vi "Untitled.vi"() -> ()   [LabVIEW 2010]
uses:
  <instrlib>/niSync/niSync.llb/niSync Initialize (IVI).vi
  glob1.vi
panel:
  out "Timing:Time Reference:Last Synchronization ID":i32
  out "Timing:Time Reference:Clock Resolution":i32
  out "Timing:Time Reference:UTC Offset Valid":bool
  out "Timing:Time Reference:UTC Offset":i32
  out "Timing:Time Reference:Time Reference Correction":dbl
  out "Timing:Time Reference:Offset from Time Reference":dbl
  out "Timing:Time Reference:Is Time Reference Present":bool
  out "Timing:Time Reference:Time Reference":i32(ring) items=["GPS", "IRIG", "PPS", "1588 Ordinary Clock", "Free Running"]
  in  "stop":bool
  out "error out":errorcluster {"code" format="%.0x"}
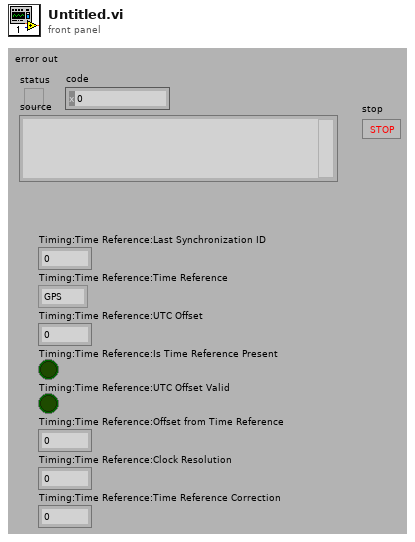
[diagram p1: front panel]
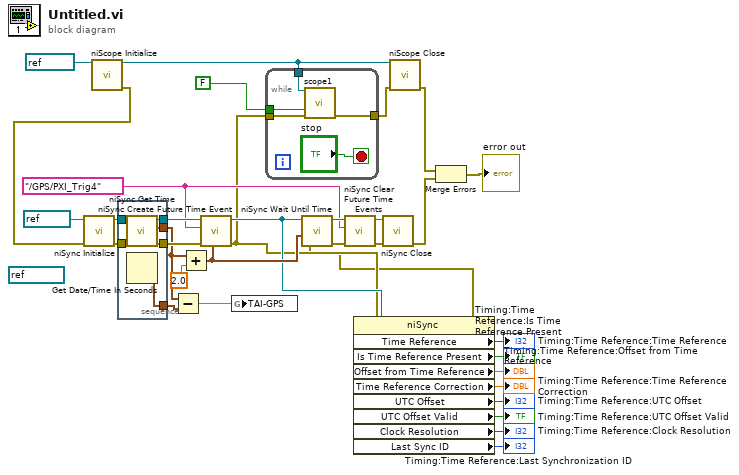
[diagram p0: block diagram]
diagram:
  w26 = tag "/GPS/PXI_Trig4" ("terminal")
  (unwired) refnum<visa-resource-name> "t6682"
  n1 = call <instrlib>:"niScope Initialize.vi"("resource name"=refnum<k15> "ADC") -> ("instrument handle"=w18:refnum<k15>, "error out"=w16:errorcluster)  [unwired: 13 in]
  n2 = call-poly <instrlib>:"niSync Initialize.vi"("error in (no error)"=w16, "resource name"=refnum<k15> "GPS") -> ("error out"=w33:errorcluster, "instrument handle out"=w34:refnum<k15>)  [unwired: 8 in]
  n3 = stacked-sequence {
    tunnel: w34 -> [w40]
    tunnel: w33 -> [w39]
    tunnel: [w38] -> w30
    tunnel: [w37] -> w29
    tunnel: [w36] -> w15
    tunnel: [w35] -> w14
    frame #0 {
      n4 = call <instrlib>:"niSync Get Time.vi"("error in (no error)"=w39, "instrument handle"=w40) -> ("error out"=w38:errorcluster, "time"=w35:timestamp, "instrument handle out"=w37:refnum<k15>)  [unwired: 5 in]
      n5 = Get Date/Time In Seconds() -> (seconds since 1Jan1904=w36:timestamp)
    }
  }
  n6 = Subtract(x=w14, y=w15) -> (x-y=w13:dbl)
  n7 = Add(x=w14, y=2.0) -> (x+y=w24:timestamp)
  n8 = call <instrlib>:"niSync Create Future Time Event.vi"("time"=w24, "error in (no error)"=w30, "terminal"=w26, "instrument handle"=w29) -> ("error out"=w10:errorcluster, "instrument handle out"=w11:refnum<k15>)  [unwired: 5 in]
  n9 = global write "glob1.vi" "TAI-GPS"(w13) -> ()
  n10 = while {
    tunnel: w10 -> [w45]
    tunnel: FALSE ("TriggerMode") -> [w44]
    tunnel: [w43] -> w19
    tunnel: w18 -> [w42]
    stop <- "stop" stop-if-true
    n11 = call "scope1.vi"("instrument handle"=w42, "TriggerMode"=w44, "error in"=w45) -> ("error out"=w43:errorcluster)  [unwired: 11 in, 1 out]
  }
  n12 = property class="niSync"(reference=w11, error in=w10) -> (error out=w9:errorcluster, "Time Reference"=→"Timing:Time Reference:Time Reference":i32, "Is Time Reference Present"=→"Timing:Time Reference:Is Time Reference Present":bool, "Offset from Time Reference"=→"Timing:Time Reference:Offset from Time Reference":dbl, "Time Reference Correction"=→"Timing:Time Reference:Time Reference Correction":dbl, "UTC Offset"=→"Timing:Time Reference:UTC Offset":i32, "UTC Offset Valid"=→"Timing:Time Reference:UTC Offset Valid":bool, "Clock Resolution"=→"Timing:Time Reference:Clock Resolution":i32, "Last Sync ID"=→"Timing:Time Reference:Last Synchronization ID":i32)  [unwired: 1 out]
  n13 = call <instrlib>:"niSync Wait Until Time.vi"("error in (no error)"=w9, "time stamp"=w24, "instrument handle"=w11) -> ("error out"=w28:errorcluster, "instrument handle out"=w27:refnum<k15>)  [unwired: 3 in]
  n14 = call <instrlib>:"niSync Clear Future Time Events.vi"("error in (no error)"=w28, "terminal"=w26, "instrument handle"=w27) -> ("error out"=w32:errorcluster, "instrument handle out"=w31:refnum<k15>)  [unwired: 6 in]
  n15 = call <instrlib>:"niSync Close.vi"("error in (no error)"=w32, "instrument handle"=w31) -> ("error out"=w23:errorcluster)  [unwired: 9 in]
  n16 = call <instrlib>:"niScope Close.vi"("instrument handle"=w18, "error in"=w19) -> ("error out"=w17:errorcluster)  [unwired: 13 in]
  n17 = Merge Errors(w17, w23) -> (→"error out":errorcluster)
